vi "FilePaths.vi"(8 "error in":errorcluster) -> (0 "error out":errorcluster, 2 "paths":T1)   [LabVIEW 2019, in "Configuration Tool.lvlib"]
doc: "This VI has the Path to the Classes and the Glyphs, Additional Behavior might be added if you want to load them from a different path. By default they are in Glyphs folder and Classes folder in the main directory"
uses:
  Configuration Tool.lvlib
  Controls/FilePaths.ctl
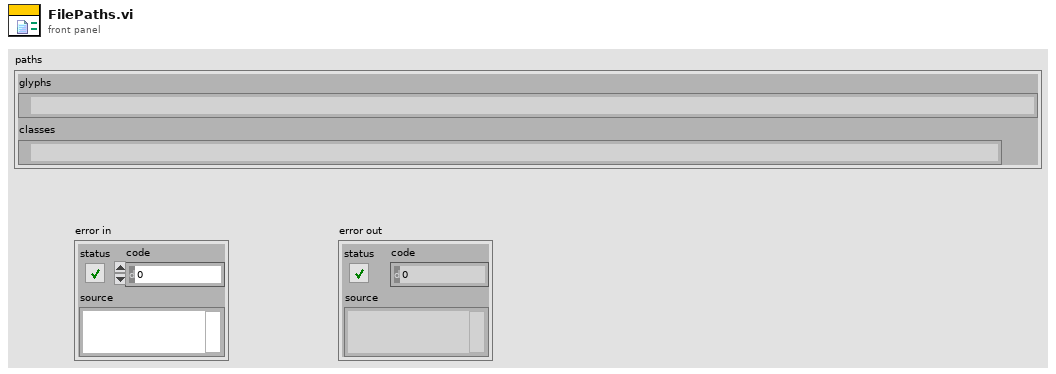
[diagram p1: front panel]
types:
  T1 = typedef "Configuration Tool.lvlib/FilePaths.ctl" = cluster{"glyphs":path, "classes":path}
  T2 = enum32{"invalid app kind", "Development System", "Run Time System", "Student Edition", "Embedded LabVIEW", "Evaluation", "Custom"}
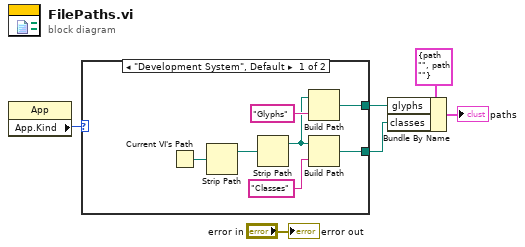
[diagram p0: block diagram]
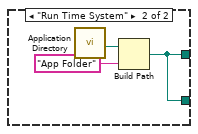
[diagram p2: hidden frame]
diagram:
  n1 = property class="App"() -> ("App.Kind"=w1:T2)  [unwired: 2 in, 2 out]
  n2 = case shown="\"Development System\", Default" w1 {
    tunnel: [w8 w14] -> w3
    tunnel: [w7 w14] -> w2
    frame "Development System", Default {
      n3 = Current VI's Path() -> (path=w11:path)
      n4 = Strip Path(path=w11) -> (stripped path=w9:path)  [unwired: 1 out]
      n5 = Strip Path(path=w9) -> (stripped path=w10:path)  [unwired: 1 out]
      n6 = Build Path(base path=w10, name or relative path="Glyphs") -> (appended path=w7:path)
      n7 = Build Path(base path=w10, name or relative path="Classes") -> (appended path=w8:path)
    }
    frame "Run Time System" {
      n8 = call <vilib>:"Application Directory.vi"() -> ("Application Directory"=w16:path)
      n9 = Build Path(base path=w16, name or relative path="App Folder") -> (appended path=w14:path)
    }
  }
  n10 = Bundle By Name(cluster=T1 {"glyphs"=path "", "classes"=path ""} ("Cluster 2"), "glyphs"=w2, "classes"=w3) -> (→"paths":T1)
  "error out" <- "error in"
